vi "ErrorCatcher.vi"(8 "error in (no error)":errorcluster, 10 "?":T1={"commandlist"="", "line"=0, "last response"="", "timeout"=0, "wait"=0, "erfolgreich"=FALSE, "next state"=enum."init", "Zustand"=enum."starting", "manual Test"=FALSE}, 11 "EMTestCWS500N in":refnum<class "EMTestCWS500N.lvclass">) -> (0 "error out":errorcluster, 3 "EMTestCWS500N out":refnum<class "EMTestCWS500N.lvclass">)   [LabVIEW 2013, in "EMTestCWS500N.lvclass"]
uses:
  EMTestCWS500N.lvclass
  Main/controls/TestData.ctl
  Main/controls/TestStates.ctl
  Main/controls/generalTestStates.ctl
  lib/EMV-Test.lvlib
panel:
  out "concatenated string":string
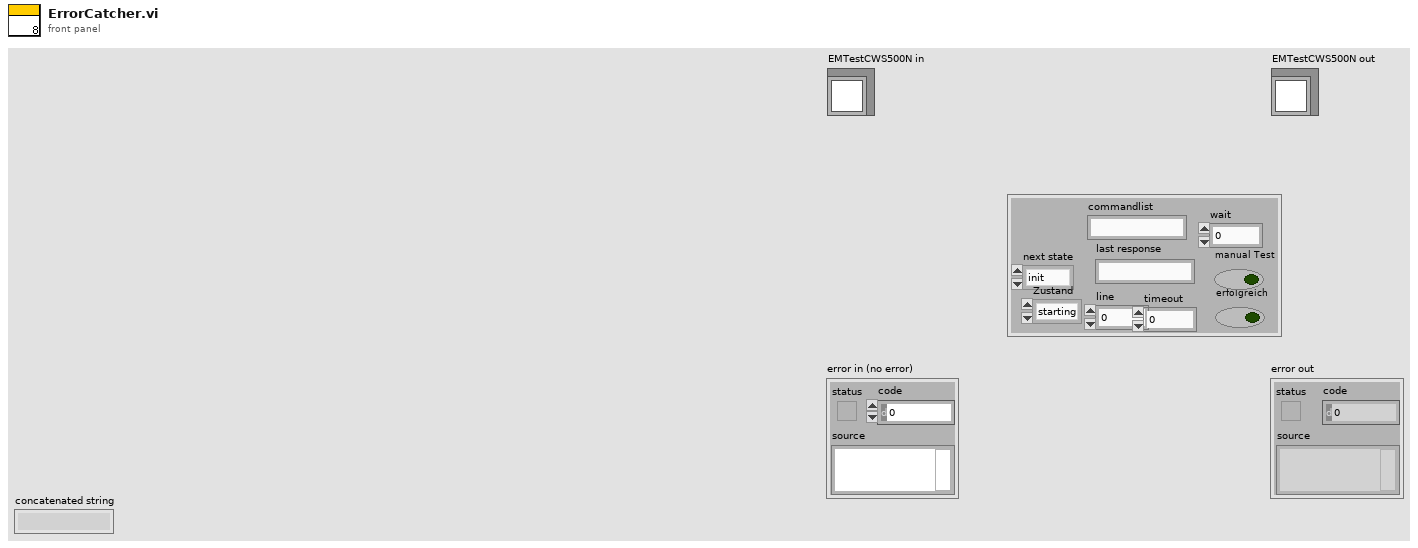
[diagram p1: front panel]
types:
  T1 = typedef "EMV-Test.lvlib/TestData.ctl" = cluster{"commandlist":string, "line":i32, "last response":string, "timeout":i32, "wait":u32, "erfolgreich":bool, "next state":T2, "Zustand":T3, "manual Test":bool}
  T2 = typedef "EMV-Test.lvlib/TestStates.ctl" = enum16{"event loop", "save Test", "Custom Action 1", "Custom Action 2", "pause", "vorgefertigter Test", "manueller Test", "respond to response", "error", "init", "start Test", "evaluate line", "wait for Response", "wait", "catch error", "close Connection", "end"}
  T3 = typedef "generalTestStates.ctl" = enum16{"paused", "starting", "waiting", "running", "finished"}
  T4 = cluster{"output string":string, "output string":string}
  T5 = cluster{"output string":string, "output string":string}[]
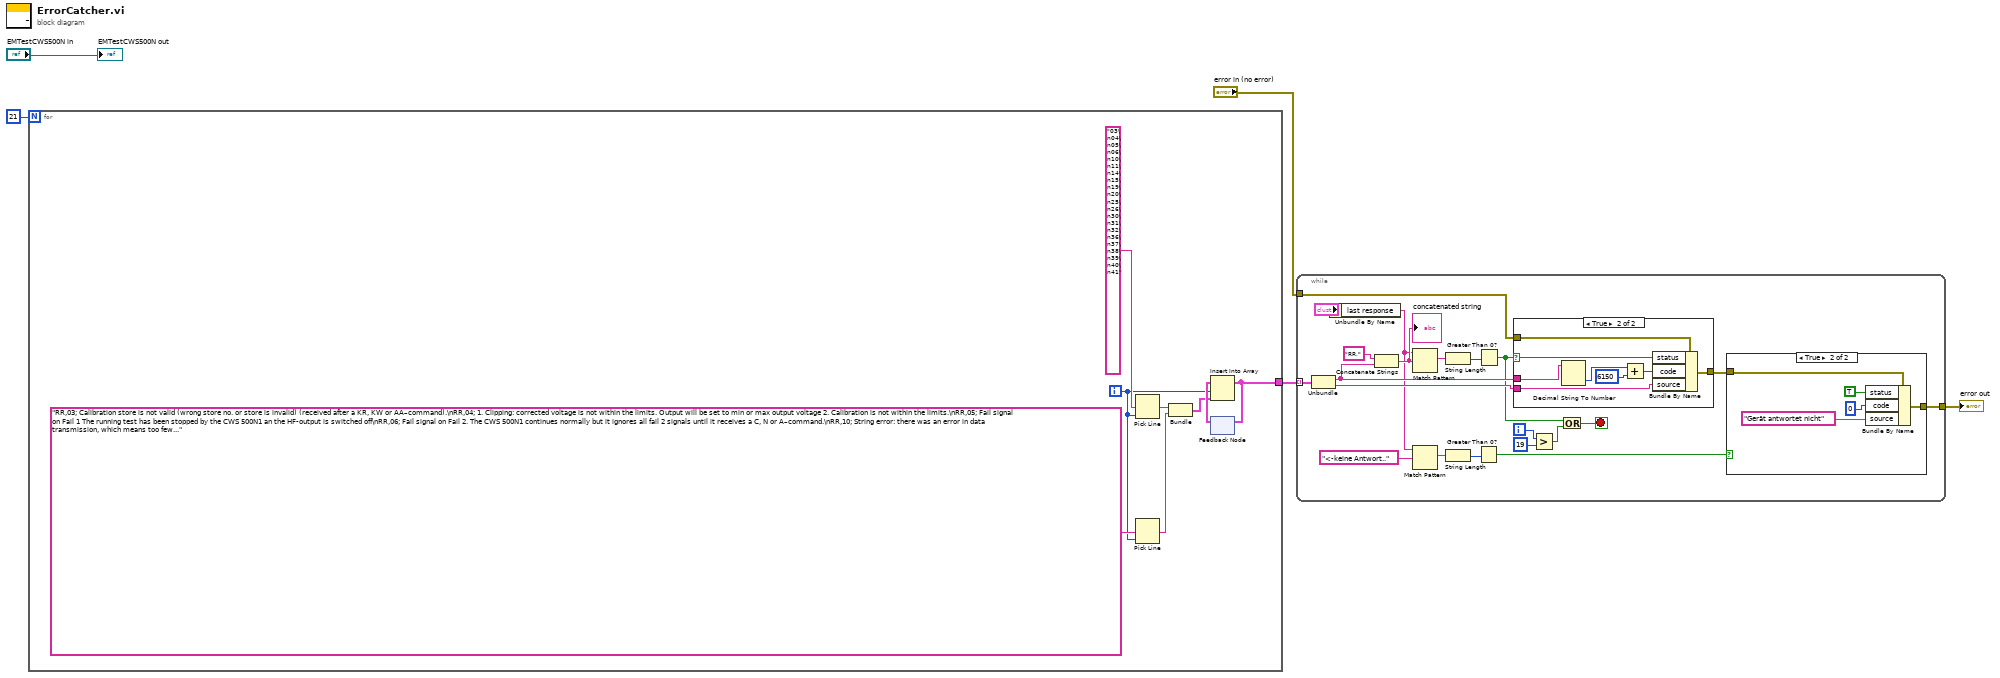
[diagram p0: block diagram]
diagram:
  n1 = for {
    N: 21 -> [_]
    tunnel: [w6] -> w5
    i -> [w8]
    n2 = Pick Line(multi-line string="03\n04\n05\n06\n10\n11\n14\n15\n19\n20\n25\n26\n30\n31\n32\n36\n37\n38\n39\n40\n41", line index=w8) -> (output string=w7:string)  [unwired: 1 in]
    n3 = Pick Line(multi-line string="RR,03; Calibration store is not valid (wrong store no. or store is invalid) (received after a KR, KW or AA–command).\nRR,04; 1. Clipping: corrected voltage is not within the limits. Output will be set to min or max output voltage 2. Calibration is not within the limits.\nRR,05; Fail signal on Fail 1 The running test has been stopped by the CWS 500N1 an the HF-output is switched off\nRR,06; Fail signal on Fail 2. The CWS 500N1 continues normally but it ignores all fail 2 signals until it receives a C, N or A–command.\nRR,10; String error: there was an error in data transmission, which means too few or too many characters or the command is not acceptable.\nRR,11; Test start is not possible or the test has been stopped because TEST ON is not switched on.\nRR,14; One or several values are limited by the CWS 500N1. The parameters are set to their minimum.\nRR,15; Check sum error. The whole command should be sent again.\nRR,19; Internal communication error. Turn off and on the CWS 500N1.\nRR,20; Not correctable limitation error. One or more parameter can not be set to its minimum.\nRR,25; The received calibration data are corrupt (Min-value or Max-value are incorrect or element-no. 265 is not set to 255) (received after a KW–command).\nRR,26; Error on internal Eeprom (write-protected, memory busy) The test routine has been finished correctly using the current monitor. •  This answer will be returned if the test has been invoked by a CN–command with a valid BCI store. parameter Description \nRR,30, V corr , max. current, corr. current; V corr : max. current: corr. current: The factor * 100 between the programmed voltage and the reduced voltage (caused by an overcurrent). The theoretical current at the programmed voltage. The measured current.\nRR,31; Answer to a AA–command if the selected BCI store doesn’t consist of valid data.\nRR,32; BCI store is not valid (the store number is invalid) (received after a KA, KB, KN or KI–command).\nRR,36; BCI store is not valid (there is no valid data in the selected BCI store or the store number is invalid)(received after a KA–command).\nRR,37; The received values for the transfer impedance of the current probe (BCI) are corrupt (Min-value or Max-value are incorrect or element-no. 49 is not set to 65535) (received after a KB–command).\nRR,38; The sent command has no function because there is no PM1000 (current monitor) built in.\nRR,39; Measuring unit not available during a running BCI test\nRR,40; Safety Circuit has been opened. Test stops\nRR,41; PM 40x protection has occured. Test stops", line index=w8) -> (output string=w11:string)  [unwired: 1 in]
    n4 = Bundle("output string"=w7, "output string"=w11) -> (w9:T4)  [unwired: 1 in]
    n5 = feedback #1() -> (w10:T5)  [unwired: 1 in]
    n6 = Insert Into Array(array=w10, index=w8, new element=w9) -> (w6:T5)
    n7 = feedback-in #1(w6) -> ()
  }
  n8 = while {
    tunnel: w5 -> [w34] mode=indexing
    tunnel: "error in (no error)" -> [w28]
    tunnel: [w16] -> w1
    i -> [w23]
    stop <- w25 stop-if-true
    n9 = Unbundle(w34) -> ("output string"=w27:string, "output string"=w30:string)
    n10 = Unbundle By Name("?") -> ("last response"=w14:string)
    n11 = Concatenate Strings("RR,", w27) -> (w29:string)
    "concatenated string" <- w29
    n12 = Match Pattern(string=w14, regular expression=w29) -> (match substring=w33:string)  [unwired: 1 in, 3 out]
    n13 = Match Pattern(string=w14, regular expression="<-keine Antwort..") -> (match substring=w20:string)  [unwired: 1 in, 3 out]
    n14 = String Length(string=w33) -> (length=w32:i32)
    n15 = String Length(string=w20) -> (length=w21:i32)
    n16 = Greater Than 0?(x=w21) -> (x > 0?=w18:bool)
    n17 = Greater Than 0?(x=w32) -> (x > 0?=w26:bool)
    n18 = case shown="True" w26 {
      selector: w26 -> [_ w48]
      tunnel: w27 -> [_ w49]
      tunnel: w30 -> [_ w47]
      tunnel: w28 -> [w41 w46]
      tunnel: [w41 w45] -> w17
      frame False {
      }
      frame True {
        n19 = Decimal String To Number(string=w49) -> (number=w43:i32)  [unwired: 2 in, 1 out]
        n20 = Add(x=w43, y=6150) -> (x+y=w42:i32)
        n21 = Bundle By Name(cluster=w46, "status"=w48, "code"=w42, "source"=w47) -> (w45:errorcluster)
      }
    }
    n22 = Greater?(x=w23, y=19) -> (0:w24:bool)
    n23 = Or(x=w26, y=w24) -> (x .or. y?=w25:bool)
    n24 = case shown="True" w18 {
      tunnel: w17 -> [w35 w39]
      tunnel: [w35 w40] -> w16
      frame False {
      }
      frame True {
        n25 = Bundle By Name(cluster=w39, "status"=TRUE, "code"=0, "source"="Gerät antwortet nicht") -> (w40:errorcluster)
      }
    }
  }
  "error out" <- w1
  "EMTestCWS500N out" <- "EMTestCWS500N in"
